vi "UART Write Bytes.vi"(7 "DataSize":i32, 9 "pWriteData":u8[](array[numeric])=array[4097 elements], 10 "Channel":u8, 11 "DevHandle":i32) -> (1 "pWriteData out":u8[](array[numeric]), 3 "function return":i32)   [LabVIEW 2010, in "usb2uart.lvlib"]
doc: "int WINAPI UART_WriteBytes(int DevHandle,unsigned char Channel,unsigned char *pWriteData,int DataSize);"
uses:
  usb2uart.lvlib
  USB2XXX.dll
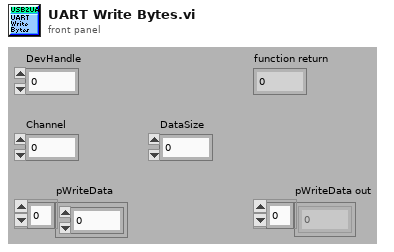
[diagram p1: front panel]
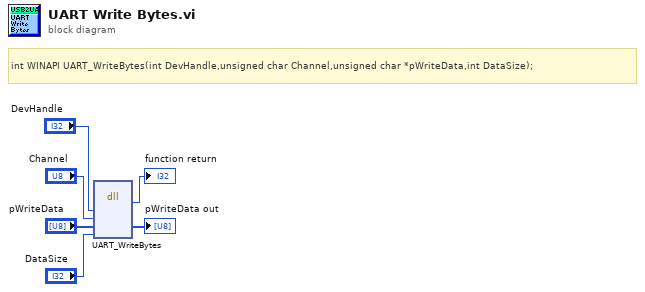
[diagram p0: block diagram]
diagram:
  # "int WINAPI UART_WriteBytes(int DevHandle,unsigned char Channel,unsigned char *pWriteData,int DataSize);"
  n1 = dll-call lib="F:/OtherWork/STM32/USB2XXX_Example/trunk/Labview/PublicFiles/USB2XXX.*" fn="UART_WriteBytes"("DevHandle"="DevHandle", "Channel"="Channel", "pWriteData"="pWriteData", "DataSize"="DataSize") -> (→"function return":i32, "pWriteData"=→"pWriteData out":u8[])  [unwired: 6 in, 2 out]
